vi "GetCameraPOSinLab2 (SubVI).vi"(8 "error in (no error)":errorcluster, 10 "Loaded array":dbl[][](array[numeric]), 11 "Refnum in":T1) -> (0 "error out":errorcluster, 1 "Image #":i32, 2 "Image coordinates in lab frame":dbl[](array[numeric]), 3 "Refnum out":T1)   [LabVIEW 2016]
uses:
  <vilib>/vision/Image Controls.llb/IMAQ Image.ctl
  <resource>/objmgr/IMAQImage.rc
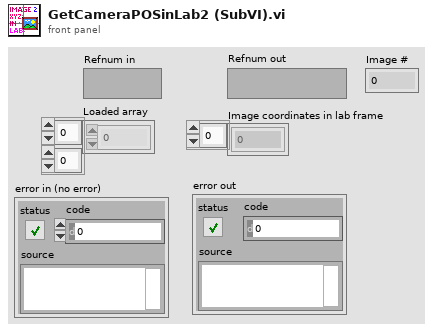
[diagram p1: front panel]
types:
  T1 = typedef "IMAQ Image.ctl" = refnum<image>
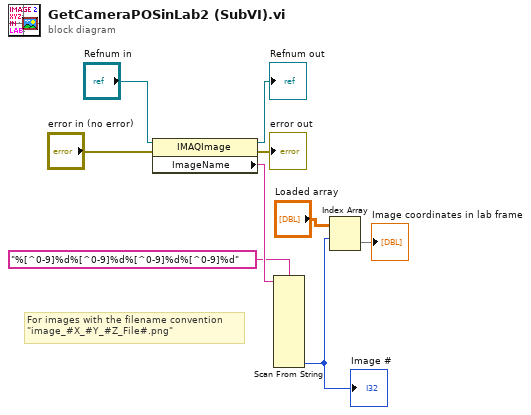
[diagram p0: block diagram]
diagram:
  # "For images with the filename convention\n\"image_#X_#Y_#Z_File#.png\""
  n1 = property class="IMAQImage"(reference="Refnum in", error in="error in (no error)") -> (reference out=→"Refnum out":T1, error out=→"error out":errorcluster, "ImageName"=w8:string)
  n2 = Scan From String(format string="%[^0-9]%d%[^0-9]%d%[^0-9]%d%[^0-9]%d", input string=w8) -> (output 8=w1:i32)  [unwired: 17 in, 3 out]
  "Image #" <- w1
  n3 = Index Array(array="Loaded array", index (row)=w1) -> (element=→"Image coordinates in lab frame":dbl[])  [unwired: 1 in]
